vi "MakeEllipse.vi"(1 "Rotation":dbl format="%.2f", 2 "Cursor 2":cluster{"Cursor X":dbl, "Cursor Y":dbl} {"Cursor Y" format="%.2f"; "Cursor X" format="%.2f"}, 3 "Cursor 1":cluster{"Cursor X":dbl, "Cursor Y":dbl} {"Cursor Y" format="%.2f"; "Cursor X" format="%.2f"}, 4 "Cursor 0":cluster{"Cursor X":dbl, "Cursor Y":dbl} {"Cursor Y" format="%.2f"; "Cursor X" format="%.2f"}) -> (0 "X-Y elipse":cluster{"x coord":dbl[], "y coord":dbl[]} {"y coord" format="%.2f"; "x coord" format="%.2f"})   [LabVIEW 2022 SP3]
uses:
  <vilib>/Analysis/NI_AALPro.lvlib
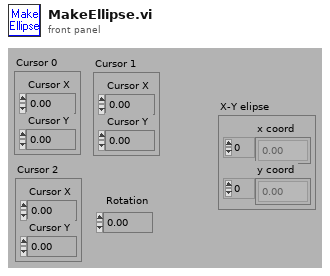
[diagram p1: front panel]
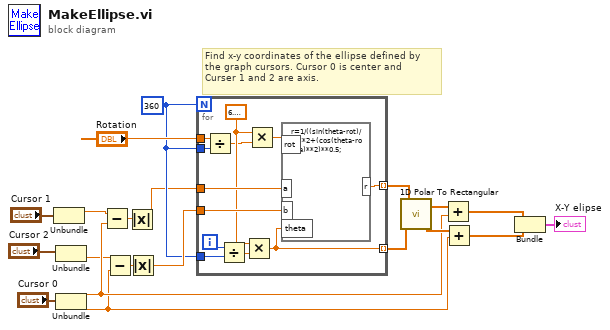
[diagram p0: block diagram]
diagram:
  w15 = 360
  # "Find x-y coordinates of the ellipse defined by\nthe graph cursors. Cursor 0 is center and\nCurser 1 and 2 are axis."
  n1 = Unbundle("Cursor 1") -> ("Cursor X"=w7:dbl)  [unwired: 1 out]
  n2 = Unbundle("Cursor 2") -> ("Cursor Y"=w6:dbl)  [unwired: 1 out]
  n3 = Unbundle("Cursor 0") -> ("Cursor X"=w11:dbl, "Cursor Y"=w10:dbl)
  n4 = Subtract(x=w7, y=w11) -> (x-y=w4:dbl)
  n5 = Subtract(x=w6, y=w10) -> (x-y=w18:dbl)
  n6 = Absolute Value(x=w4) -> (abs(x)=w3:dbl)
  n7 = Absolute Value(x=w18) -> (abs(x)=w19:dbl)
  n8 = for {
    N: w15 -> [_]
    tunnel: "Rotation" -> [w24]
    tunnel: w3 -> [w32]
    tunnel: w19 -> [w31]
    tunnel: w15 -> [w28]
    tunnel: [w26] -> w14 mode=indexing
    tunnel: [w27] -> w13 mode=indexing
    tunnel: w15 -> [w21]
    i -> [w29]
    w23 = 6.283185307179586
    n9 = Divide(x=w24, y=w21) -> (x/y=w22:dbl)
    n10 = Divide(x=w29, y=w28) -> (x/y=w30:dbl)
    n11 = Multiply(x=w23, y=w30) -> (x*y=w27:dbl)
    n12 = Multiply(x=w23, y=w22) -> (x*y=w25:dbl)
    n13 = formula code="r=1/((sin(theta-rot)/b)**2+(cos(theta-rot)/a)**2)**0.5;"("rot"=w25, "a"=w32, "b"=w31, "theta"=w27) -> ("r"=w26:dbl)
  }
  n14 = call <vilib>:"1D Polar To Rectangular.vi"("Magnitude"=w14, "Phase"=w13) -> ("X"=w16:dbl[], "Y"=w17:dbl[])  [unwired: 1 out]
  n15 = Add(x=w16, y=w11) -> (x+y=w1:dbl[])
  n16 = Add(x=w17, y=w10) -> (x+y=w2:dbl[])
  n17 = Bundle(w1, w2) -> (→"X-Y elipse":cluster{dbl[], dbl[]})  [unwired: 1 out]
